vi "G# - GetObjectStatus.vi"() -> ()   [LabVIEW 2020]
doc: "Get Object Status\n\nThis example demonstrates the use of the G#Object support method GetObjectStatus.vi."
uses:
  MyDemoClass_class/MyDemoClass.lvclass
  vi.lib/addons/_AddQ/G#Object/G#Object.lvclass
panel:
  out "ToString":string[](array[string])
  in  "simple info (F)":bool
  out "# of users?":i32
  out "last user":bool
  out "class name":string
  out "counter?":bool
  out "object name":string
  out "not a refnum?":bool
  out "# of objects":i32
  out "all object names":string[](array[string])
  out "full class name":string
  in  "Object Index":i32
  out "error out":errorcluster
  # "Get Object Status\nThis example demonstrates the use of the G#Object support method GetObjectStatus.vi."
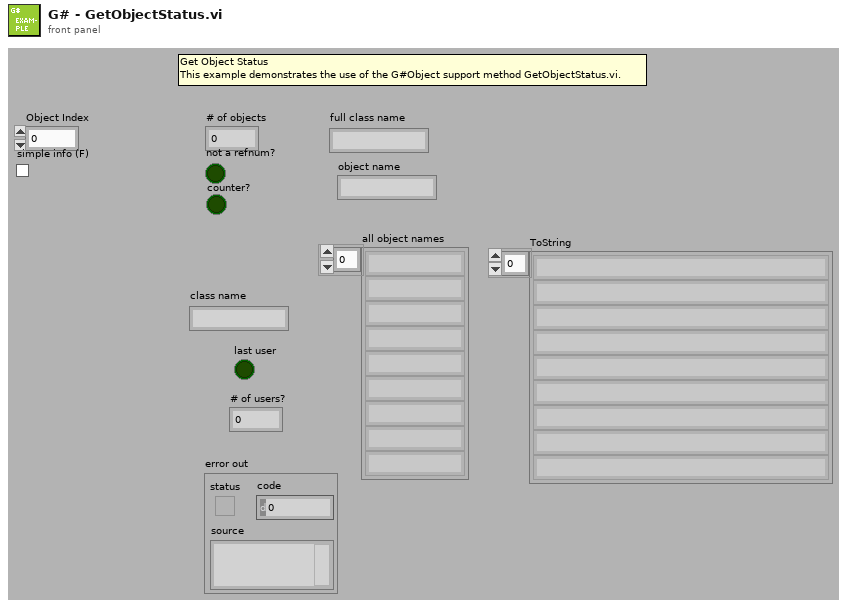
[diagram p1: front panel]
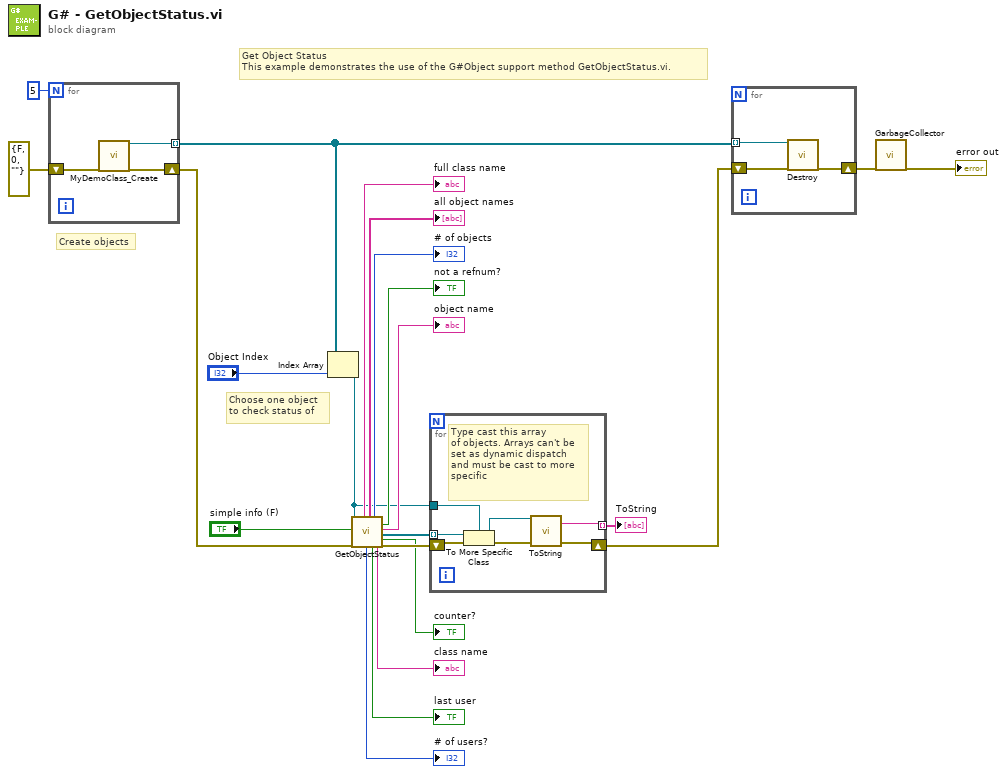
[diagram p0: block diagram]
diagram:
  # "Choose one object\nto check status of"
  # "Create objects"
  # "Get Object Status\nThis example demonstrates the use of the G#Object support method GetObjectStatus.vi."
  n1 = for {
    N: 5 -> [_]
    shift-right: [w25] -> w22
    shift-left: errorcluster {"status"=FALSE, "code"=0, "source"=""} ("error out") -> [w24]
    tunnel: [w23] -> w19 mode=indexing
    n2 = call "MyDemoClass_Create.vi"("error in (no error)"=w24) -> ("reference out"=w23:refnum<class "MyDemoClass.lvclass">, "error out"=w25:errorcluster)  [unwired: 17 in]
  }
  n3 = Index Array(array=w19, index="Object Index") -> (element=w8:refnum<class "MyDemoClass.lvclass">)
  n4 = call-dynamic "GetObjectStatus.vi"("reference in"=w8, "simple info (F)"="simple info (F)", "error in (no error)"=w22) -> ("full class name"=→"full class name":string, "# of users?"=→"# of users?":i32, "all object names"=→"all object names":string[], "last user"=→"last user":bool, "# of objects"=→"# of objects":i32, "class name"=→"class name":string, "not a refnum?"=→"not a refnum?":bool, "object name"=→"object name":string, "all refs out"=w9:refnum<class "G#Object.lvclass">[], "counter?"=→"counter?":bool, "error out"=w10:errorcluster)  [unwired: 5 in, 1 out]
  n5 = for {
    shift-right: [w27] -> w7
    shift-left: w10 -> [w32]
    tunnel: w9 -> [w31] mode=indexing
    tunnel: w8 -> [w30]
    tunnel: [w26] -> w1 mode=indexing
    # "Type cast this array\nof objects. Arrays can't be\nset as dynamic dispatch\nand must be cast to more\nspecific"
    n6 = To More Specific Class(target class=w30, reference=w31, error in=w32) -> (specific class reference=w29:refnum<class "MyDemoClass.lvclass">, error out=w28:errorcluster)
    n7 = call-dynamic "ToString.vi"("reference in"=w29, "error in (no error)"=w28) -> ("string"=w26:string, "error out"=w27:errorcluster)  [unwired: 15 in, 1 out]
  }
  "ToString" <- w1
  n8 = for {
    shift-right: [w33] -> w18
    shift-left: w7 -> [w35]
    tunnel: w19 -> [w34] mode=indexing
    n9 = call-dynamic "Destroy.vi"("reference in"=w34, "error in (no error)"=w35) -> ("error out"=w33:errorcluster)  [unwired: 16 in, 1 out]
  }
  n10 = call "GarbageCollector.vi"("error in (no error)"=w18) -> ("error out"=→"error out":errorcluster)  [unwired: 16 in, 2 out]
